vi "BatchModeTest.vi"() -> ()   [LabVIEW 2020]
uses:
  <vilib>/httpClient/LabVIEWHTTPClient.lvlib
panel:
  out "batch-mode-pulses-remaining":i32
  out "LaserOn?":bool
  in  "Batch Size":dbl
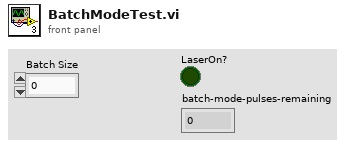
[diagram p1: front panel]
types:
  T1 = typedef "LabVIEWHTTPClient.lvlib/ClientHandle.ctl" = refnum<k1>
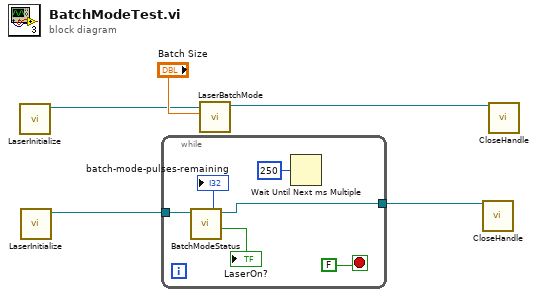
[diagram p0: block diagram]
diagram:
  n1 = call "LaserInitialize.vi"() -> ("client handle out"=w3:T1)  [unwired: 11 in]
  n2 = call "LaserInitialize.vi"() -> ("client handle out"=w1:T1)  [unwired: 11 in]
  n3 = while {
    tunnel: w1 -> [w11]
    tunnel: [w9] -> w2
    stop <- FALSE stop-if-true
    n4 = call "BatchModeStatus.vi"("client handle in"=w11) -> ("LaserOn?"=→"LaserOn?":bool, "batch-mode-pulses-remaining"=→"batch-mode-pulses-remaining":i32, "client handle out"=w9:T1)  [unwired: 8 in]
    n5 = Wait Until Next ms Multiple(millisecond multiple=u32 250) -> ()  [unwired: 1 out]
  }
  n6 = call "LaserBatchMode.vi"("Batch Size"="Batch Size", "client handle in"=w3) -> ("client handle out"=w5:T1)  [unwired: 9 in]
  n7 = call <vilib>:"CloseHandle.vi"("client handle"=w2) -> ()  [unwired: 14 in, 1 out]
  n8 = call <vilib>:"CloseHandle.vi"("client handle"=w5) -> ()  [unwired: 14 in, 1 out]
